vi "MM in Range.vi"(8 "Right Position":dbl=4099.0, 9 "Right Setpoint":dbl=4096.0, 10 "Left position":dbl=3980.0, 11 "Left Setpoint":dbl=4096.0) -> (2 "\"Done with step\" enough":bool=TRUE)   [LabVIEW 2018]
panel:
  in  "Acceptable Range":dbl=150.0
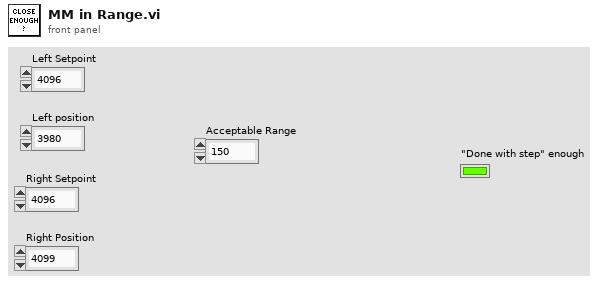
[diagram p1: front panel]
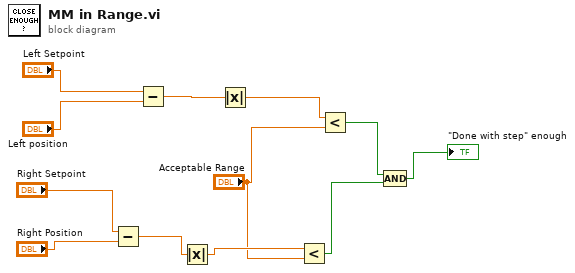
[diagram p0: block diagram]
diagram:
  n1 = Subtract(x="Right Setpoint", y="Right Position") -> (x-y=w3:dbl)
  n2 = Subtract(x="Left Setpoint", y="Left position") -> (x-y=w5:dbl)
  n3 = Absolute Value(x=w3) -> (abs(x)=w2:dbl)
  n4 = Absolute Value(x=w5) -> (abs(x)=w4:dbl)
  n5 = Less?(x=w2, y="Acceptable Range") -> (x < y?=w7:bool)
  n6 = Less?(x=w4, y="Acceptable Range") -> (x < y?=w6:bool)
  n7 = Compound Arithmetic op=AND(w6, w7) -> (→"\"Done with step\" enough":bool)
